vi "RunWithRecording.vi"(8 "error in (no error)":errorcluster, 11 "UI_Interaction_Manager in":refnum<class "UI_Interaction_Manager.lvclass">) -> (0 "error out":errorcluster, 2 "ControlValueUpdates[]":T1[](array[typedef]), 3 "UI_Interaction_Manager out":refnum<class "UI_Interaction_Manager.lvclass">)   [LabVIEW 2011, in "UI_Interaction_Manager.lvclass"]
uses:
  UI_Interaction_Manager.lvclass
  TypeDefs/ControlValueUpdate.ctl
  UI_Interaction_Manager.lvclass/UI_Interaction_Manager.ctl
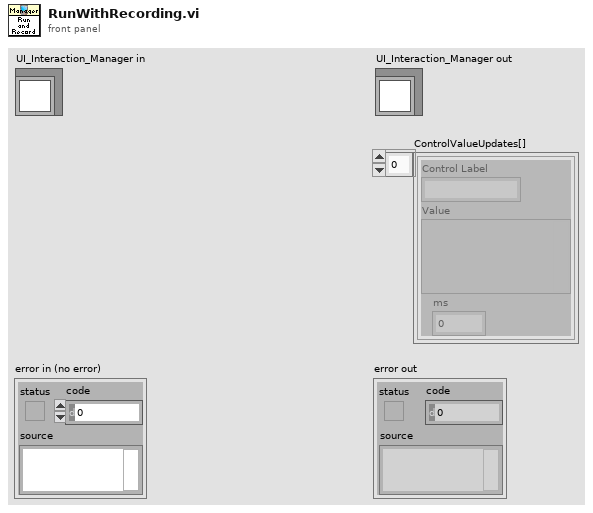
[diagram p1: front panel]
types:
  T1 = typedef "UI_Interaction_Manager.lvclass/ControlValueUpdate.ctl" = cluster{"Control Label":string, "Value":variant, "ms":u32}
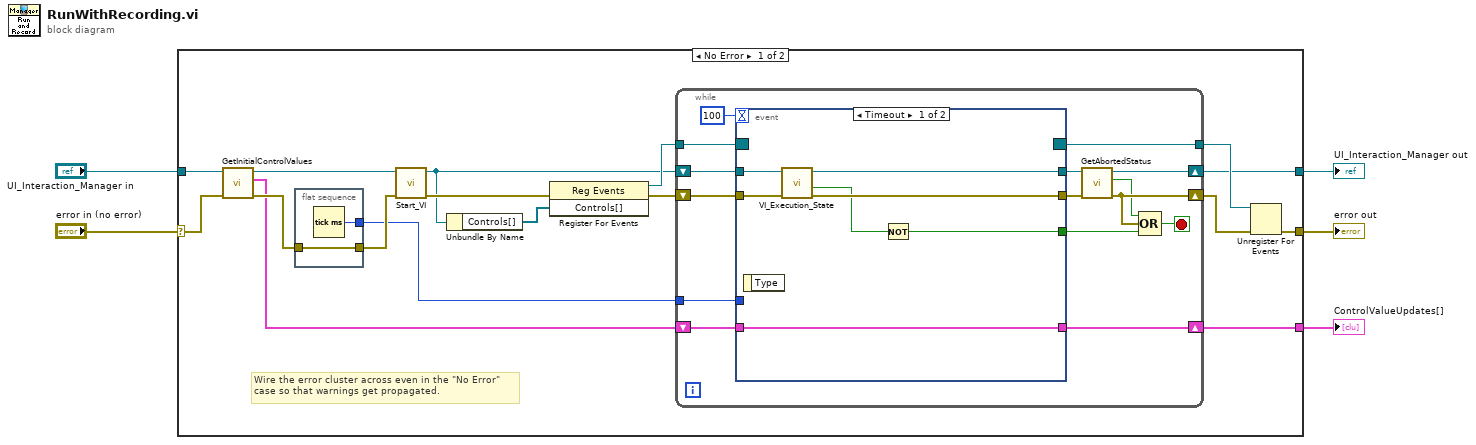
[diagram p0: block diagram]
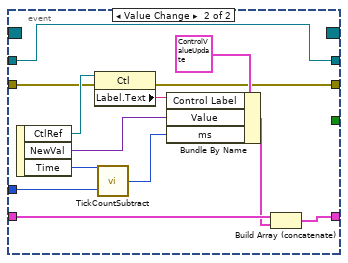
[diagram p2: hidden frame]
diagram:
  n1 = case shown="No Error" "error in (no error)" {
    selector: "error in (no error)" -> [w9 w61]
    tunnel: [w14 w61] -> w4
    tunnel: [w13 w60] -> w2
    tunnel: "UI_Interaction_Manager in" -> [w8 w60]
    tunnel: [w10 _] -> w1
    frame No Error {
      # "Wire the error cluster across even in the \"No Error\"\ncase so that warnings get propagated."
      n2 = call "GetInitialControlValues.vi"("error in (no error)"=w9, "UI_Interaction_Manager in"=w8) -> ("error out"=w22:errorcluster, "ControlValueUpdates[]"=w11:T1[], "UI_Interaction_Manager out"=w20:refnum<class "UI_Interaction_Manager.lvclass">)  [unwired: 7 in]
      n3 = flat-sequence {
        tunnel: [w59] -> w12
        tunnel: w22 -> [w58]
        tunnel: [w58] -> w21
        frame #0 {
          n4 = Tick Count (ms)() -> (millisecond timer value=w59:u32)
        }
      }
      n5 = call "Start_VI.vi"("error in (no error)"=w21, "UI_Interaction_Manager in"=w20) -> ("error out"=w19:errorcluster, "UI_Interaction_Manager out"=w6:refnum<class "UI_Interaction_Manager.lvclass">)  [unwired: 8 in]
      n6 = Unbundle By Name(w6) -> ("Controls[]"=w7:refnum<vi>[])
      n7 = register-events(error in=w19, w7) -> (reference out=w17:refnum<event-registration>, error out=w18:errorcluster)  [unwired: 1 in]
      n8 = while {
        shift-right: [w28] -> w13
        shift-left: w6 -> [w36]
        shift-right: [w25] -> w15
        shift-left: w18 -> [w35]
        shift-right: [w33] -> w10
        shift-left: w11 -> [w34]
        tunnel: w17 -> [w32]
        tunnel: [w31] -> w16
        tunnel: w12 -> [w23]
        stop <- w26 stop-if-true
        n9 = event shown="[0] Timeout" {
          selector: w32 -> [_ _]
          dyn-events: [_ _] -> w31
          timeout: 100 -> [_ _]
          tunnel: [w39 _] -> w27
          tunnel: w36 -> [w43 w48]
          tunnel: w35 -> [w42 w56]
          tunnel: [w41 w48] -> w30
          tunnel: [w40 w52] -> w29
          tunnel: w34 -> [w44 w51]
          tunnel: [w44 w49] -> w33
          tunnel: w23 -> [_ w46]
          event Timeout {
            n10 = event-data() -> ()  [unwired: 1 in, 1 out]
            n11 = call "VI_Execution_State.vi"("error in (no error)"=w42, "UI_Interaction_Manager in"=w43) -> ("error out"=w40:errorcluster, "Running?"=w38:bool, "UI_Interaction_Manager out"=w41:refnum<class "UI_Interaction_Manager.lvclass">)  [unwired: 6 in, 1 out]
            n12 = Not(x=w38) -> (.not. x?=w39:bool)
          }
          event Value Change {
            n13 = event-data() -> ("CtlRef"=w57:refnum<vi>, "NewVal"=w54:variant, "Time"=w47:u32)  [unwired: 1 in]
            n14 = property class="Ctl"(reference=w57, error in=w56) -> (error out=w52:errorcluster, "Label.Text"=w55:string)  [unwired: 1 out]
            n15 = call "TickCountSubtract.vi"("Old Time"=w46, "New Time"=w47) -> ("Time Change"=w45:u32)
            n16 = Bundle By Name(cluster=T1 {"Control Label"="", "Value"=variant, "ms"=0}, "Control Label"=w55, "Value"=w54, "ms"=w45) -> (w50:T1)
            n17 = Build Array (concatenate)(w51, w50) -> (w49:T1[])
          }
        }
        n18 = call "GetAbortedStatus.vi"("error in (no error)"=w29, "UI_Interaction_Manager in"=w30) -> ("error out"=w25:errorcluster, "Aborted?"=w24:bool, "UI_Interaction_Manager out"=w28:refnum<class "UI_Interaction_Manager.lvclass">)  [unwired: 7 in]
        n19 = Compound Arithmetic op=OR(w24, w25, w27) -> (w26:bool)
      }
      n20 = Unregister For Events(event registration refnum=w16, error in=w15) -> (error out=w14:errorcluster)
    }
    frame Error {
    }
  }
  "error out" <- w4
  "UI_Interaction_Manager out" <- w2
  "ControlValueUpdates[]" <- w1
